vi "SHGetFolderPath.vi"(0 "error in (no error)":errorcluster, 1 "Return Current Path:F / Default Path:T (F)":bool, 3 "CSIDL":T2(ring), 4 "Create directory if it does not exist (F)":bool) -> (2 "error out":errorcluster, 5 "Path":path)   [LabVIEW 2020]
doc: "SHGetFolderPath.vi Version 1.0\nThis VI calls shfolder.dll to find windows system directories. The valid inputs are listed below. There are four missing values (x0C to x0F) which the input enum lists as DUMMY1-DUMMY4. If any of these are called the VI returns <Not A Path>, and an error. The same error is returned if the input is theoretically meaningful, but not in the current system (e.g. one of the directories only present on RISC installations). If the input is technically valid, but the directory does not exist, shfolder returns an empty path, so the VI returns <Not A Path> and an error.\n\nThe error handling system (SHFolderPath Append Error Codes.vi, SHFolderPath Error Enumeration.ctl, and SHFolderPath Insert Error.vi) is that provided as freeware by David A. Moore (www.mooregoodideas.com) which allows the combination of many subprojects while avoiding error code overlaps.\n\nSHFolderPath.vi is freeware, B.J. Treves Brown, DIAS, UMIST, Manchester UK \nhttp://www.in.umist.ac.uk/PRF/bernard/labview.html\n\nCSIDL_DESKTOP 0 {desktop}\nCSIDL_INTERNET 1 Internet Explorer (icon on desktop)\nCSIDL_PROGRAMS 2 Start Menu\\Programs\nCSIDL_CONTROLS 3 My Computer\\Control Panel\nCSIDL_PRINTERS 4 My Computer\\Printers\nCSIDL_PERSONAL 5 My Documents\nCSIDL_FAVORITES 6 {user name}\\Favourites\nCSIDL_STARTUP 7 Start Menu\\Programs\\Startup\nCSIDL_RECENT 8 {user name}\\Recent\nCSIDL_SENDTO 9 {user name}\\SendTo\nCSIDL_BITBUCKET A {desktop}\\Recycle Bin\nCSIDL_STARTMENU B {user name}\\Start Menu\nCSIDL_DESKTOPDIRECTORY 10 {user name}\\Desktop\nCSIDL_DRIVES 11 My Computer\nCSIDL_NETWORK 12 Network Neighborhood\nCSIDL_NETHOOD 13 {user name}\\nethood\nCSIDL_FONTS 14 windows\\fonts\nCSIDL_TEMPLATES 15\nCSIDL_COMMON_STARTMENU 16 All Users\\Start Menu\nCSIDL_COMMON_PROGRAMS 17 All Users\\Programs\nCSIDL_COMMON_STARTUP 18 All Users\\Startup\nCSIDL_COMMON_DESKTOPDIRECTORY 19 All Users\\Desktop\nCSIDL_APPDATA 1A {user name}\\Application Data\nCSIDL_PRINTHOOD 1B {user name}\\PrintHood\nCSIDL_LOCAL_APPDATA 1C {user name}\\Local Settings\\\n _Application Data (non roaming)\nCSIDL_ALTSTARTUP 1D non localized startup\nCSIDL_COMMON_ALTSTARTUP 1E non localized common startup\nCSIDL_COMMON_FAVORITES 1F\nCSIDL_INTERNET_CACHE 20\nCSIDL_COOKIES 21\nCSIDL_HISTORY 22\nCSIDL_COMMON_APPDATA 23 All Users\\Application Data\nCSIDL_WINDOWS 24 GetWindowsDirectory()\nCSIDL_SYSTEM 25 GetSystemDirectory()\nCSIDL_PROGRAM_FILES 26 C:\\Program Files\nCSIDL_MYPICTURES 27 C:\\Program Files\\My Pictures\nCSIDL_PROFILE 28 USERPROFILE\nCSIDL_SYSTEMX86 29 x86 system directory on RISC\nCSIDL_PROGRAM_FILESX86 2A x86 C:\\Program Files on RISC\nCSIDL_PROGRAM_FILES_COMMON 2B C:\\Program Files\\Common\nCSIDL_PROGRAM_FILES_COMMONX86 2C x86 Program Files\\Common on RISC\nCSIDL_COMMON_TEMPLATES 2D All Users\\Templates\nCSIDL_COMMON_DOCUMENTS 2E All Users\\Documents\nCSIDL_COMMON_ADMINTOOLS 2F All Users\\Start Menu\\ _\n Programs\\Administrative Tools\nCSIDL_ADMINTOOLS 30 {user name}\\Start Menu _\n \\Programs\\Administrative Tools"
uses:
  SHGetFolderPath Errors.ctl
  shfolder.dll
panel:
  in  "SHGetFolderPath Error Enumeration":T1
  # "CSIDL                        Hex   Description\n                             Value\nCSIDL_DESKTOP                   0  {desktop}\nCSIDL_INTERNET                  1  Internet Explorer (icon on desktop)\nCSIDL_PROGRAMS                  2  Start Menu\\Programs\nCSIDL_CONTROLS                  3  My Computer\\Control Panel\nCSIDL_PRINTERS                  4  My Computer\\Printers\nCSIDL_PERSONAL                  5  My Documents\nCSIDL_FAVORITES                 6  {user name}\\Favourites\nCSIDL_STARTUP                   7  Start Menu\\Programs\\Startup\nCSIDL_RECENT                    8  {user name}\\Recent\nCSIDL_SENDTO                    9  {user name}\\SendTo\nCSIDL_BITBUCKET                 A  {desktop}\\Recycle Bin\nCSIDL_STARTMENU                 B  {user name}\\Start Menu\nCSIDL_DESKTOPDIRECTORY         10  {user name}\\Desktop\nCSIDL_DRIVES                   11  My Computer\nCSIDL_NETWORK                  12  Network Neighborhood\nCSIDL_NETHOOD                  13  {user name}\\nethood\nCSIDL_FONTS                    14  windows\\fonts\nCSIDL_TEMPLATES                15\nCSIDL_COMMON_STARTMENU         16  All Users\\Start Menu\nCSIDL_COMMON_PROGRAMS          17  All Users\\Programs\nCSIDL_COMMON_STARTUP           18  All Users\\Startup\nCSIDL_COMMON_DESKTOPDIRECTORY  19  All Users\\Desktop\nCSIDL_APPDATA                  1A  {user name}\\Application Data\nCSIDL_PRINTHOOD                1B  {user name}\\PrintHood\nCSIDL_LOCAL_APPDATA            1C  {user name}\\Local Settings\\\n                                   _Application Data (non roaming)\nCSIDL_ALTSTARTUP               1D  non localized startup\nCSIDL_COMMON_ALTSTARTUP        1E  non localized common startup\nCSIDL_COMMON_FAVORITES         1F\nCSIDL_INTERNET_CACHE           20\nCSIDL_COOKIES                  21\nCSIDL_HISTORY                  22\nCSIDL_COMMON_APPDATA           23  All Users\\Application Data\nCSIDL_WINDOWS                  24  GetWindowsDirectory()\nCSIDL_SYSTEM                   25  GetSystemDirectory()\nCSIDL_PROGRAM_FILES            26  C:\\Program Files\nCSIDL_MYPICTURES               27  C:\\Program Files\\My Pictures\nCSIDL_PROFILE                  28  USERPROFILE\nCSIDL_SYSTEMX86                29  x86 system directory on RISC\nCSIDL_PROGRAM_FILESX86         2A  x86 C:\\Program Files on RISC\nCSIDL_PROGRAM_FILES_COMMON     2B  C:\\Program Files\\Common\nCSIDL_PROGRAM_FILES_COMMONX86  2C  x86 Program Files\\Common on RISC\nCSIDL_COMMON_TEMPLATES         2D  All Users\\Templates\nCSIDL_COMMON_DOCUMENTS         2E  All Users\\Documents\nCSIDL_COMMON_ADMINTOOLS        2F  All Users\\Start Menu\\ _\n                                   Programs\\Administrative Tools\nCSIDL_ADMINTOOLS               30  {user name}\\Start Menu _"
  # "SHGetFolderPath.vi Version 1.0\nWritten by:\nB.J. Treves Brown\nDIAS, UMIST\nManchester \nUK\n4th April 2001\nhttp://www.in.umist.ac.uk/PRF/bernard/labview.html\n\nBased on the examples in:\nQ252652 - HOWTO: Use the SHGetFolderPath Function from Visual Basic\nhttp://support.microsoft.com/support/kb/articles/Q252/6/52.asp\nby Microsoft Inc.\n\nError handling VIs by David A. Moore (www.mooregoodideas.com)"
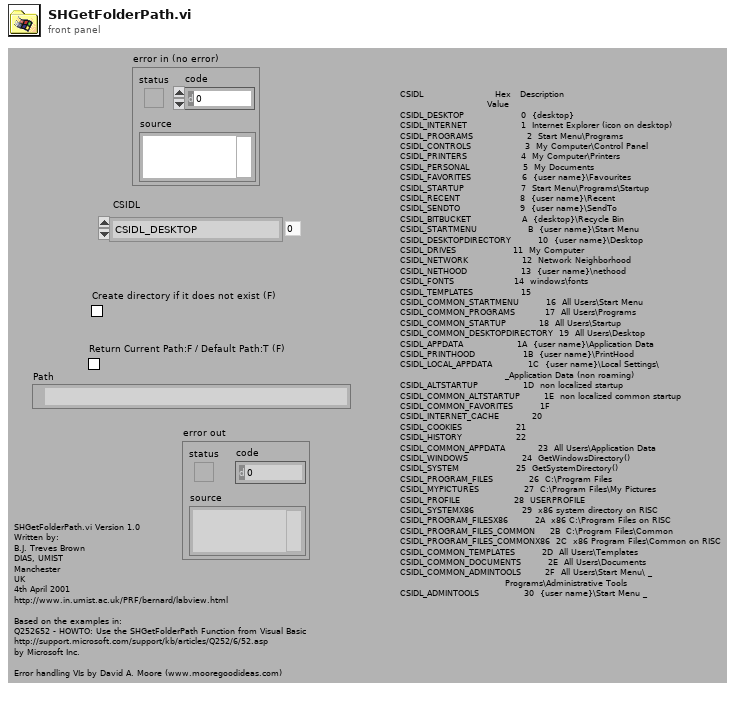
[diagram p1: front panel]
types:
  T1 = typedef "SHGetFolderPath Errors.ctl" = enum16{"The Folder is valid, but does not exist", "An invalid folder ID was specified", "Unrecognized Result from SHFolderPath call"}
  T2 = enum16{"CSIDL_DESKTOP", "CSIDL_INTERNET", "CSIDL_PROGRAMS", "CSIDL_CONTROLS", "CSIDL_PRINTERS\n", "CSIDL_PERSONAL", "CSIDL_FAVORITES", "CSIDL_STARTUP", "CSIDL_RECENT", "CSIDL_SENDTO", "CSIDL_BITBUCKET", "CSIDL_STARTMENU", "DUMMY1", "DUMMY2", "DUMMY3", "DUMMY4", "CSIDL_DESKTOPDIRECTORY", "CSIDL_DRIVES", "CSIDL_NETWORK", "CSIDL_NETHOOD", "CSIDL_FONTS", "CSIDL_TEMPLATES", "CSIDL_COMMON_STARTMENU", "CSIDL_COMMON_PROGRAMS", "CSIDL_COMMON_STARTUP", "CSIDL_COMMON_DESKTOPDIRECTORY", "CSIDL_APPDATA", "CSIDL_PRINTHOOD", "CSIDL_LOCAL_APPDATA", "CSIDL_ALTSTARTUP", "CSIDL_COMMON_ALTSTARTUP", "CSIDL_COMMON_FAVORITES", "CSIDL_INTERNET_CACHE", "CSIDL_COOKIES", "CSIDL_HISTORY", "CSIDL_COMMON_APPDATA", "CSIDL_WINDOWS", "CSIDL_SYSTEM", "CSIDL_PROGRAM_FILES", "CSIDL_MYPICTURES", "CSIDL_PROFILE", "CSIDL_SYSTEMX86", "CSIDL_PROGRAM_FILESX86", "CSIDL_PROGRAM_FILES_COMMON", "CSIDL_PROGRAM_FILES_COMMONX86", "CSIDL_COMMON_TEMPLATES", "CSIDL_COMMON_DOCUMENTS", "CSIDL_COMMON_ADMINTOOLS", "CSIDL_ADMINTOOLS"}
  T3 = cluster{bool, "Error Code Base":i32, "Call Chain for calling VI":string}
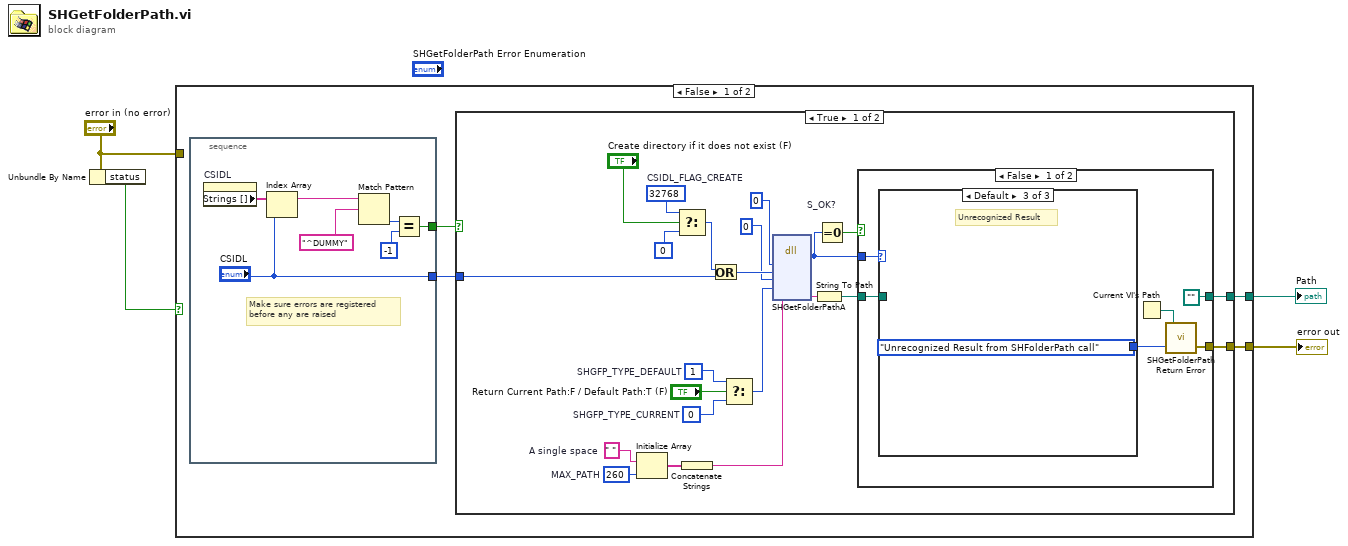
[diagram p0: block diagram]
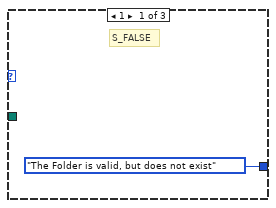
[diagram p2: hidden frame]
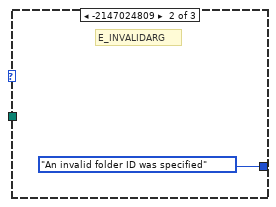
[diagram p3: hidden frame]
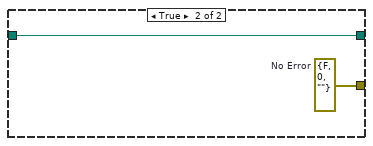
[diagram p4: hidden frame]
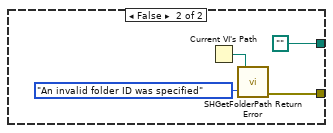
[diagram p5: hidden frame]
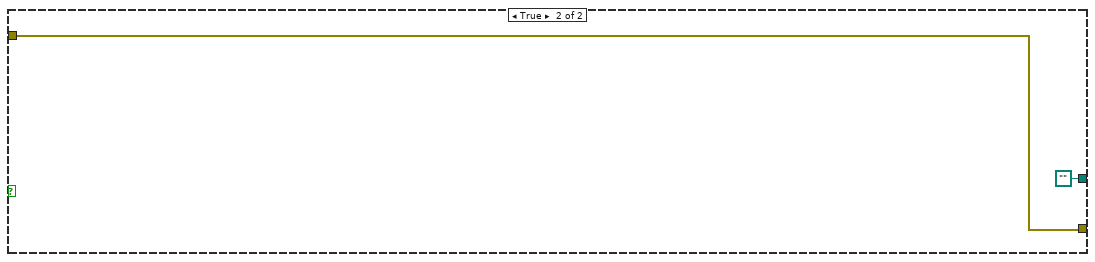
[diagram p6: hidden frame]
diagram:
  n1 = Unbundle By Name("error in (no error)") -> ("status"=w2:bool)
  n2 = case shown="False" w2 {
    tunnel: [w6 w54] -> w4
    tunnel: [w5 path ""] -> w3
    tunnel: "error in (no error)" -> [_ w54]
    frame False {
      n3 = stacked-sequence {
        tunnel: ["CSIDL"] -> w8
        tunnel: [w9] -> w7
        frame #0 {
          # "Make sure errors are registered before any are raised"
          n4 = property on="CSIDL" class="Enum (strict)"() -> ("Strings []"=w15:string[])  [unwired: 2 in, 2 out]
          n5 = Index Array(array=w15, index="CSIDL") -> (element=w14:string)
          n6 = Match Pattern(string=w14, regular expression="^DUMMY") -> (offset past match=w12:i32)  [unwired: 1 in, 3 out]
          n7 = Equal?(x=w12, y=-1) -> (x = y?=w9:bool)
        }
      }
      n8 = case shown="True" w7 {
        tunnel: w8 -> [w21 _]
        tunnel: [w19 path ""] -> w5
        tunnel: [w16 w50] -> w6
        frame True {
          w26 = " "  # A single space
          w27 = 260  # MAX_PATH
          w30 = u32 1  # SHGFP_TYPE_DEFAULT
          w29 = u32 0  # SHGFP_TYPE_CURRENT
          w36 = 32768  # CSIDL_FLAG_CREATE
          n9 = Initialize Array(w26, w27) -> (w25:string[])
          n10 = Select(t=w36, s="Create directory if it does not exist (F)", f=0) -> (s? t:f=w22:i32)
          n11 = Concatenate Strings(w25) -> (w24:string)
          n12 = Or(x=w22, y=w21) -> (x .or. y?=w33:i32)
          n13 = Select(t=w30, s="Return Current Path:F / Default Path:T (F)", f=w29) -> (s? t:f=w28:u32)
          n14 = dll-call lib="shfolder.dll" fn="SHGetFolderPathA"("hwndOwner"=u32 0, "nFolder"=w33, "hToken"=u32 0, "dwFlags"=w28, "pszPath"=w24) -> (w17:u32, "pszPath"=w23:string)  [unwired: 7 in, 2 out]
          n15 = String To Path(string=w23) -> (path=w20:path)
          n16 = Equal To 0? "S_OK?"(x=w17) -> (x = 0?=w18:bool)
          n17 = case shown="False" w18 {
            tunnel: w20 -> [w43 w48]
            tunnel: [path "" w48] -> w19
            tunnel: w17 -> [w42 _]
            tunnel: [w38 w47] -> w16
            frame False {
              n18 = case shown="Default" w42 {
                tunnel: w43 -> [_ _ _]
                tunnel: [SHGetFolderPath_Errors."The Folder is valid, but does not exist" ("SHGetFolderPath Error Enumeration") SHGetFolderPath_Errors."An invalid folder ID was specified" ("SHGetFolderPath Error Enumeration") SHGetFolderPath_Errors."Unrecognized Result from SHFolderPath call" ("SHGetFolderPath Error Enumeration")] -> w40
                frame 1 {
                  # "S_FALSE"
                }
                frame -2147024809 {
                  # "E_INVALIDARG"
                }
                frame Default {
                  # "Unrecognized Result"
                }
              }
              n19 = Current VI's Path() -> (path=w39:path)
              n20 = call "SHGetFolderPath Return Error.vi"("SHGetFolderPath Error Enumeration"=w40, "Path"=w39) -> ("error out"=w38:errorcluster)  [unwired: 1 in]
            }
            frame True {
              w47 = T3 {FALSE, "Error Code Base"=0, "Call Chain for calling VI"=""}  # No Error
            }
          }
        }
        frame False {
          n21 = Current VI's Path() -> (path=w51:path)
          n22 = call "SHGetFolderPath Return Error.vi"("SHGetFolderPath Error Enumeration"=SHGetFolderPath_Errors."An invalid folder ID was specified", "Path"=w51) -> ("error out"=w50:errorcluster)  [unwired: 1 in]
        }
      }
    }
    frame True {
    }
  }
  "error out" <- w4
  "Path" <- w3
